vi "util.file.vars.path-parser.vi"(8 "error in (no error)":errorcluster, 9 "allowDialogs?(False)":bool, 10 "location (PROCEDURE_DIR)":T1, 11 "Proc name":string) -> (0 "error out":errorcluster, 1 "cancelled":bool, 3 "selected path":path)   [LabVIEW 2024]
uses:
  controls/typePathSelector.ctl
  <vilib>/Utility/error.llb/Clear Errors.vi
  <vilib>/Utility/libraryn.llb/Create Directory Recursive.vi
panel:
  # "May be prefixed with base folder"
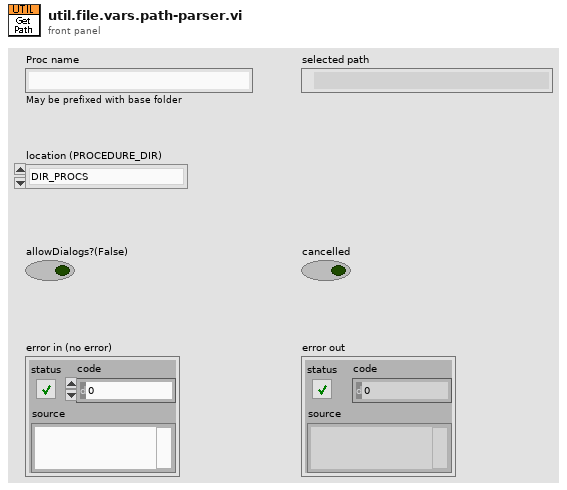
[diagram p1: front panel]
types:
  T1 = typedef "typePathSelector.ctl" = enum16{"DIR_PROCS", "DIR_CONFIG", "DIR_TEMPLATE", "DIR_IO_FILE", "DIR_RECORD", "DIR_LOG", "DIR_RUNTIME", "DIR_PRESET", "DIR_INI"}
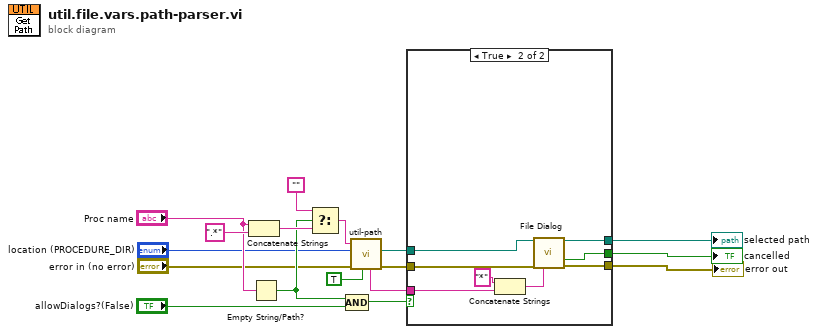
[diagram p0: block diagram]
diagram:
  n1 = Concatenate Strings("Proc name", ".*") -> (w12:string)
  n2 = Empty String/Path?(string/path="Proc name") -> (empty?=w11:bool)
  n3 = Select(t="", s=w11, f=w12) -> (s? t:f=w13:string)
  n4 = Compound Arithmetic op=AND(w11, "allowDialogs?(False)") -> (w8:bool)
  n5 = call "util-path.vi"("Create Folders?(F)"=TRUE, "error in"="error in (no error)", "Selected Folder (PROCS)"="location (PROCEDURE_DIR)", "append path (ie. folder\\filename.*)"=w13) -> ("error out"=w6:errorcluster, "SelectedPath"=w5:path, ".extension (.prc)"=w7:string)  [unwired: 3 in, 2 out]
  n6 = case shown="True" w8 {
    tunnel: [w18 w27] -> w1
    tunnel: [_ w26] -> w3
    tunnel: [w19 w25] -> w17
    tunnel: w5 -> [w19 w24]
    tunnel: w6 -> [w18 w23]
    tunnel: w7 -> [_ w22]
    frame False {
    }
    frame True {
      n7 = Concatenate Strings("*" ("string"), w22) -> (w21:string)
      n8 = call "File Dialog"("start path"=w24, "error in"=w23, "pattern (all files)"=w21) -> ("selected path"=w25:path, "cancelled"=w26:bool, "error out"=w27:errorcluster)  [unwired: 9 in, 1 out]
    }
  }
  "selected path" <- w17
  "cancelled" <- w3
  "error out" <- w1
